vi "Read sTA.vi"(8 "error in (no error)":errorcluster, 11 "DAM0404D in":refnum<class "DAM0404D.lvclass">) -> (0 "error out":errorcluster, 3 "DAM0404D out":refnum<class "DAM0404D.lvclass">)   [LabVIEW 2016, in "DAM0404D.lvlib" / "DAM0404D.lvclass"]
uses:
  DAM0404D.lvclass
  DAM0404D.lvclass/DAM0404D.ctl
  <vilib>/Plasmionique/MB Master/MB Master.lvlib
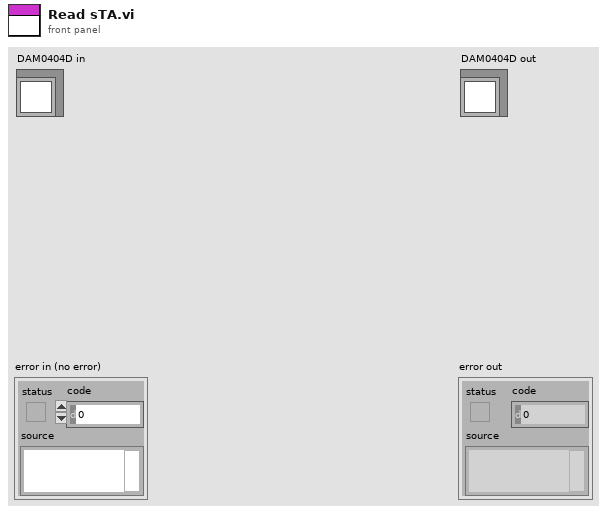
[diagram p1: front panel]
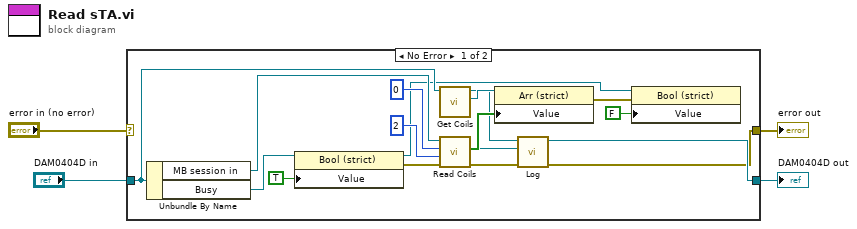
[diagram p0: block diagram]
diagram:
  n1 = case shown="No Error" "error in (no error)" {
    selector: "error in (no error)" -> [_ w23]
    tunnel: [w6 w23] -> w3
    tunnel: [w8 w22] -> w1
    tunnel: "DAM0404D in" -> [w16 w22]
    frame No Error {
      n2 = Unbundle By Name(w16) -> ("MB session in"=w21:refnum<class "MB_Master.lvclass">, "Busy"=w15:refnum<vi>)
      n3 = property class="Bool (strict)"(reference=w15, "Value"=TRUE) -> (reference out=w13:refnum<vi>, error out=w10:errorcluster)  [unwired: 1 in]
      n4 = call "Get Coils.vi"("DAM0404D in"=w16) -> ("Coils"=w18:refnum<vi>, "DAM0404D out"=w9:refnum<class "DAM0404D.lvclass">)  [unwired: 9 in]
      n5 = call <vilib>:"Read Coils.vi"("error in (no error)"=w10, "quantity"=u16 2, "starting address"=u16 0, "MB session in"=w21) -> ("error out"=w7:errorcluster, "Coils"=w17:bool[], "MB session out"=w5:refnum<class "MB_Master.lvclass">)  [unwired: 5 in]
      n6 = property class="Arr (strict)"(reference=w18, "Value"=w17) -> (error out=w11:errorcluster)  [unwired: 1 in, 1 out]
      n7 = call "Log.vi"("error in (no error)"=w7, "MB session in"=w5, "DAM0404D in"=w9) -> ("error out"=w6:errorcluster, "DAM0404D out"=w8:refnum<class "DAM0404D.lvclass">)  [unwired: 7 in]
      n8 = property class="Bool (strict)"(reference=w13, error in=w11, "Value"=FALSE) -> ()  [unwired: 2 out]
    }
    frame Error {
    }
  }
  "error out" <- w3
  "DAM0404D out" <- w1
